vi "Create Config.vi"(8 "error in (no error)":errorcluster, 10 "Elements":refnum<class "Config Element.lvclass">[](array[class]), 11 "Config Storage in":refnum<class "Config Storage.lvclass">) -> (0 "error out":errorcluster, 2 "Config":refnum<class "Config Manager.lvclass">, 3 "Config Storage out":refnum<class "Config Storage.lvclass">)   [LabVIEW 2020, in "CDM-Config.lvlib" / "Config Storage.lvclass"]
uses:
  Config Storage.lvclass
  Config Element/Config Element.lvclass
  Config Manager/Config Manager.lvclass
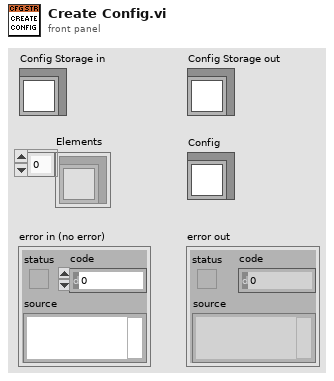
[diagram p1: front panel]
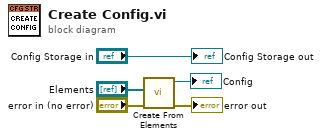
[diagram p0: block diagram]
diagram:
  n1 = call "Create From Elements.vi"("error in (no error)"="error in (no error)", "Elements"="Elements") -> ("error out"=→"error out":errorcluster, "Config Manager out"=→"Config":refnum<class "Config Manager.lvclass">)  [unwired: 8 in]
  "Config Storage out" <- "Config Storage in"
